vi "Basic Write Data.vi"(6 "chip select  (1st chip)":enum16{"1st chip", "2nd chip"}(ring), 8 "error in (no error)":errorcluster, 10 "character code":u8=97 format="%.0x", 11 "cluster of private data in":T1={"FPGA VI Reference"=refnum, "device index"=0, "screen size"=enum."8x1", "font size"=enum."5x8", "auto wrap"=FALSE, "alignment"=enum."None", "number of line"=enum."2 lines", "shift 0"=0, "entry mode 0"=enum."increment & no shift", "shift 1"=0, "entry mode 1"=enum."increment & no shift"}) -> (0 "error out":errorcluster, 3 "cluster of private data out":T1={"FPGA VI Reference"=refnum, "device index"=0, "screen size"=enum."8x1", "font size"=enum."5x8", "auto wrap"=FALSE, "alignment"=enum."None", "number of line"=enum."2 lines", "shift 0"=0, "entry mode 0"=enum."increment & no shift", "shift 1"=0, "entry mode 1"=enum."increment & no shift"})   [LabVIEW 2017, in "HD44780.lvclass"]
uses:
  HD44780.lvclass
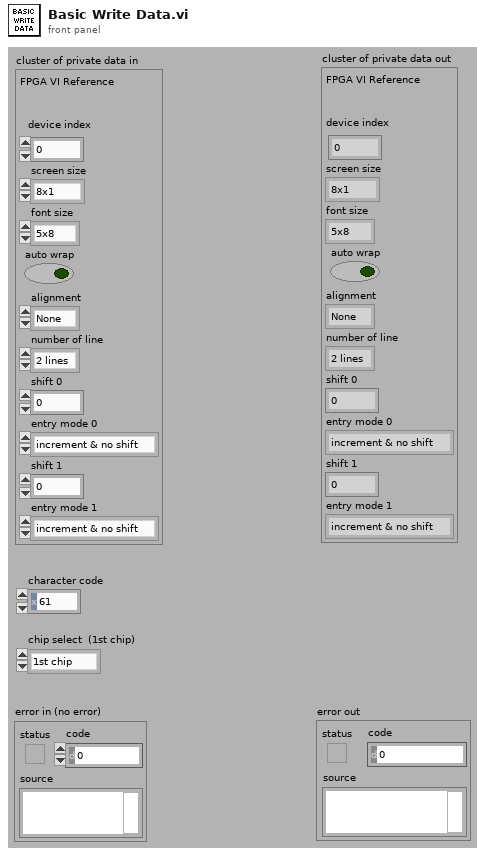
[diagram p1: front panel]
types:
  T1 = cluster{"FPGA VI Reference":refnum<k20>, "device index":i8, "screen size":enum8{"8x1", "8x2", "12x4", "16x1", "16x2", "16x4", "20x1", "20x2", "20x4", "24x1", "24x2", "40x2", "40x4"}, "font size":enum8{"5x8", "5x10"}, "auto wrap":bool, "alignment":enum16{"None", "Left", "Center", "Right"}, "number of line":enum8{"1 line", "2 lines"}, "shift 0":i8, "entry mode 0":enum8{"increment & no shift", "increment & shift", "decrement & no shift", "decrement & shift"}, "shift 1":i8, "entry mode 1":enum8{"increment & no shift", "increment & shift", "decrement & no shift", "decrement & shift"}}
  T2 = enum8{"increment & no shift", "increment & shift", "decrement & no shift", "decrement & shift"}
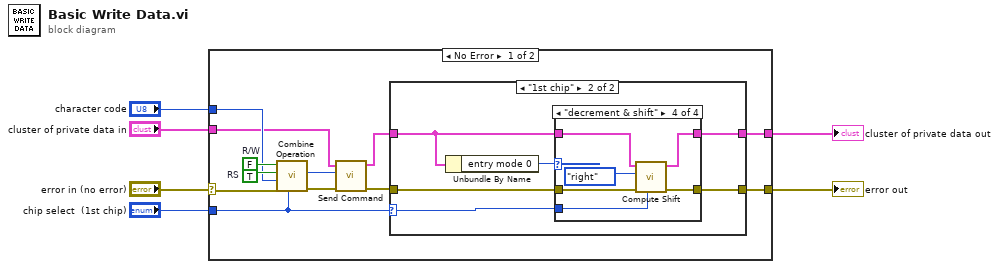
[diagram p0: block diagram]
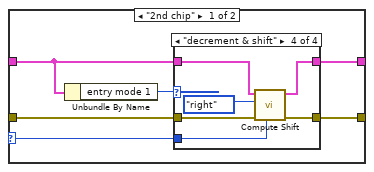
[diagram p2: hidden frame]
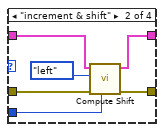
[diagram p4: hidden frame]
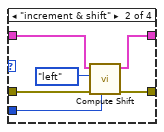
[diagram p7: hidden frame]
diagram:
  n1 = case shown="No Error" "error in (no error)" {
    selector: "error in (no error)" -> [w8 w64]
    tunnel: [w13 w63] -> w6
    tunnel: [w12 w64] -> w5
    tunnel: "character code" -> [w11 _]
    tunnel: "cluster of private data in" -> [w10 w63]
    tunnel: "chip select  (1st chip)" -> [w7 _]
    frame No Error {
      w17 = TRUE  # RS
      w18 = FALSE  # R/W
      n2 = call "Combine Operation.vi"("chip select  (1st chip)"=w7, "error in (no error)"=w8, "cmd/data"=w11, "RS"=w17, "R/W"=w18) -> ("error out"=w16:errorcluster, "output"=w14:u32)  [unwired: 5 in]
      n3 = call "Send Command.vi"("error in (no error)"=w16, "operation"=w14, "cluster of private data in"=w10) -> ("error out"=w15:errorcluster, "cluster of private data out"=w9:T1)  [unwired: 6 in, 1 out]
      n4 = case shown="\"1st chip\"" w7 {
        selector: w7 -> [w23 w45]
        tunnel: w9 -> [w19 w41]
        tunnel: [w22 w44] -> w13
        tunnel: w15 -> [w21 w43]
        tunnel: [w20 w42] -> w12
        frame "2nd chip" {
          n5 = Unbundle By Name(w19) -> ("entry mode 1"=w24:T2)
          n6 = case shown="\"decrement & shift\"" w24 {
            tunnel: w19 -> [w26 w28 w34 w36]
            tunnel: [w26 w27 w34 w35] -> w22
            tunnel: w23 -> [_ w31 _ w40]
            tunnel: w21 -> [w25 w30 w33 w38]
            tunnel: [w25 w29 w33 w37] -> w20
            frame "increment & no shift", Default {
            }
            frame "increment & shift" {
              n7 = call "Compute Shift.vi"("chip select  (1st chip)"=w31, "error in (no error)"=w30, "shift direction"=enum16{"left", "right"}."left", "cluster of private data in"=w28) -> ("error out"=w29:errorcluster, "cluster of private data out"=w27:T1)  [unwired: 6 in]
            }
            frame "decrement & no shift" {
            }
            frame "decrement & shift" {
              n8 = call "Compute Shift.vi"("chip select  (1st chip)"=w40, "error in (no error)"=w38, "shift direction"=enum16{"left", "right"}."right", "cluster of private data in"=w36) -> ("error out"=w37:errorcluster, "cluster of private data out"=w35:T1)  [unwired: 6 in]
            }
          }
        }
        frame "1st chip" {
          n9 = Unbundle By Name(w41) -> ("entry mode 0"=w46:T2)
          n10 = case shown="\"decrement & shift\"" w46 {
            tunnel: w41 -> [w48 w50 w56 w58]
            tunnel: [w48 w49 w56 w57] -> w44
            tunnel: w45 -> [_ w53 _ w62]
            tunnel: w43 -> [w47 w52 w55 w60]
            tunnel: [w47 w51 w55 w59] -> w42
            frame "increment & no shift", Default {
            }
            frame "increment & shift" {
              n11 = call "Compute Shift.vi"("chip select  (1st chip)"=w53, "error in (no error)"=w52, "shift direction"=enum16{"left", "right"}."left", "cluster of private data in"=w50) -> ("error out"=w51:errorcluster, "cluster of private data out"=w49:T1)  [unwired: 6 in]
            }
            frame "decrement & no shift" {
            }
            frame "decrement & shift" {
              n12 = call "Compute Shift.vi"("chip select  (1st chip)"=w62, "error in (no error)"=w60, "shift direction"=enum16{"left", "right"}."right", "cluster of private data in"=w58) -> ("error out"=w59:errorcluster, "cluster of private data out"=w57:T1)  [unwired: 6 in]
            }
          }
        }
      }
    }
    frame Error {
    }
  }
  "cluster of private data out" <- w6
  "error out" <- w5
